vi "HGdynamicTest.vi"(0 "SceneObject in":refnum<vi>, 1 "data (can be any type)":string, 5 "Child 3":refnum<vi>, 7 "Angle Target":T1, 9 "Child 2":refnum<vi>, 11 "Child":refnum<vi>, 12 "Direction":enum16{"CW", "CCW"}(ring), 13 "Child 4":refnum<vi>) -> (2 "Angle":sgl, 3 "x*y":dbl, 4 "SceneNode out":refnum<vi>(3d-picture), 6 "number":dbl, 8 "number 2":dbl, 10 "number 3":dbl, 14 "number 5":dbl, 15 "number 4":dbl)   [LabVIEW 2020]
uses:
  Angle Target NEW type def.ctl
  <vilib>/picture/3D Picture Control/NI_3D Picture Control.lvlib
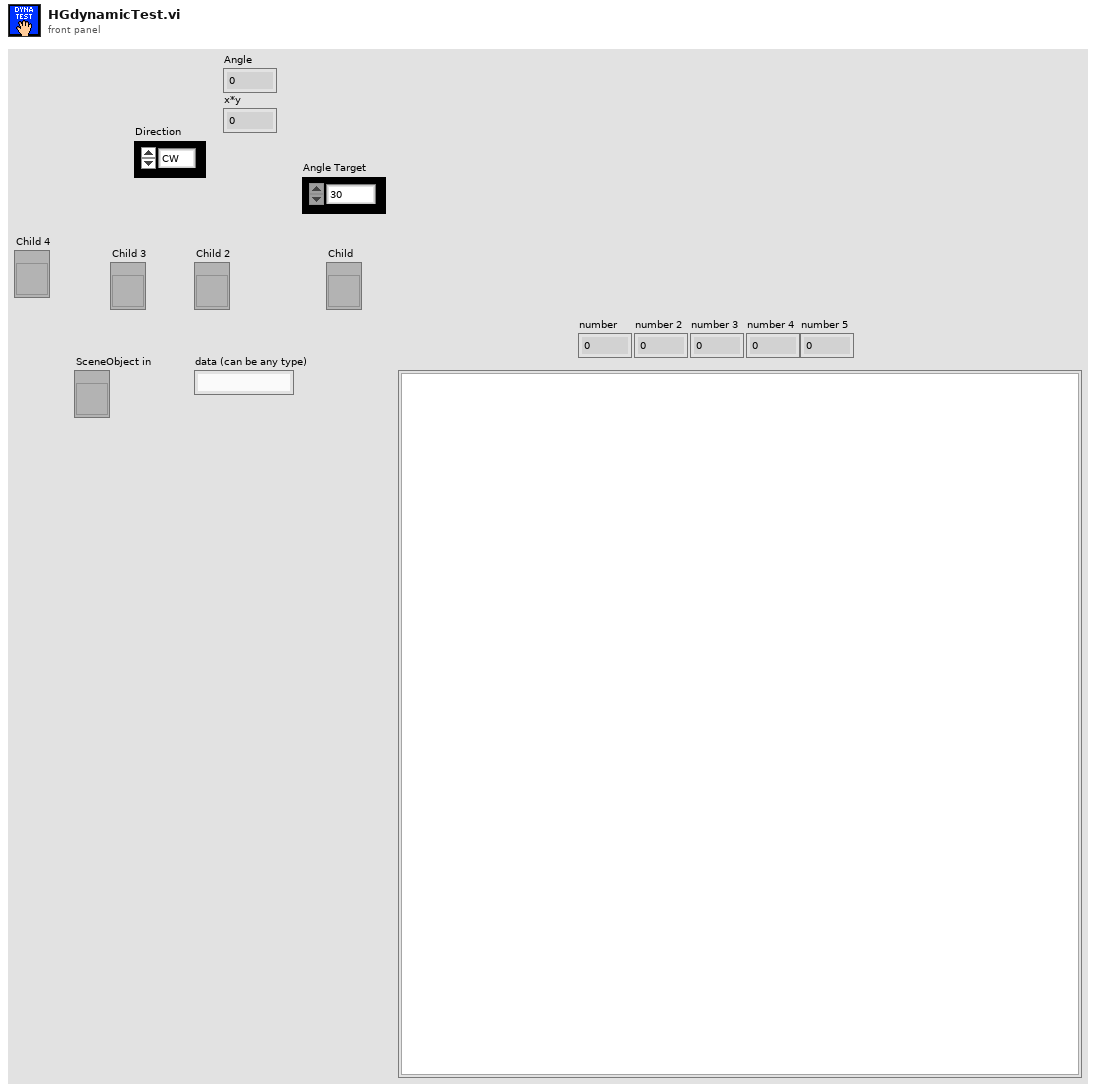
[diagram p1: front panel]
types:
  T1 = typedef "Angle Target NEW type def.ctl" = enum16{"30", "45", "60", "75", "90"}
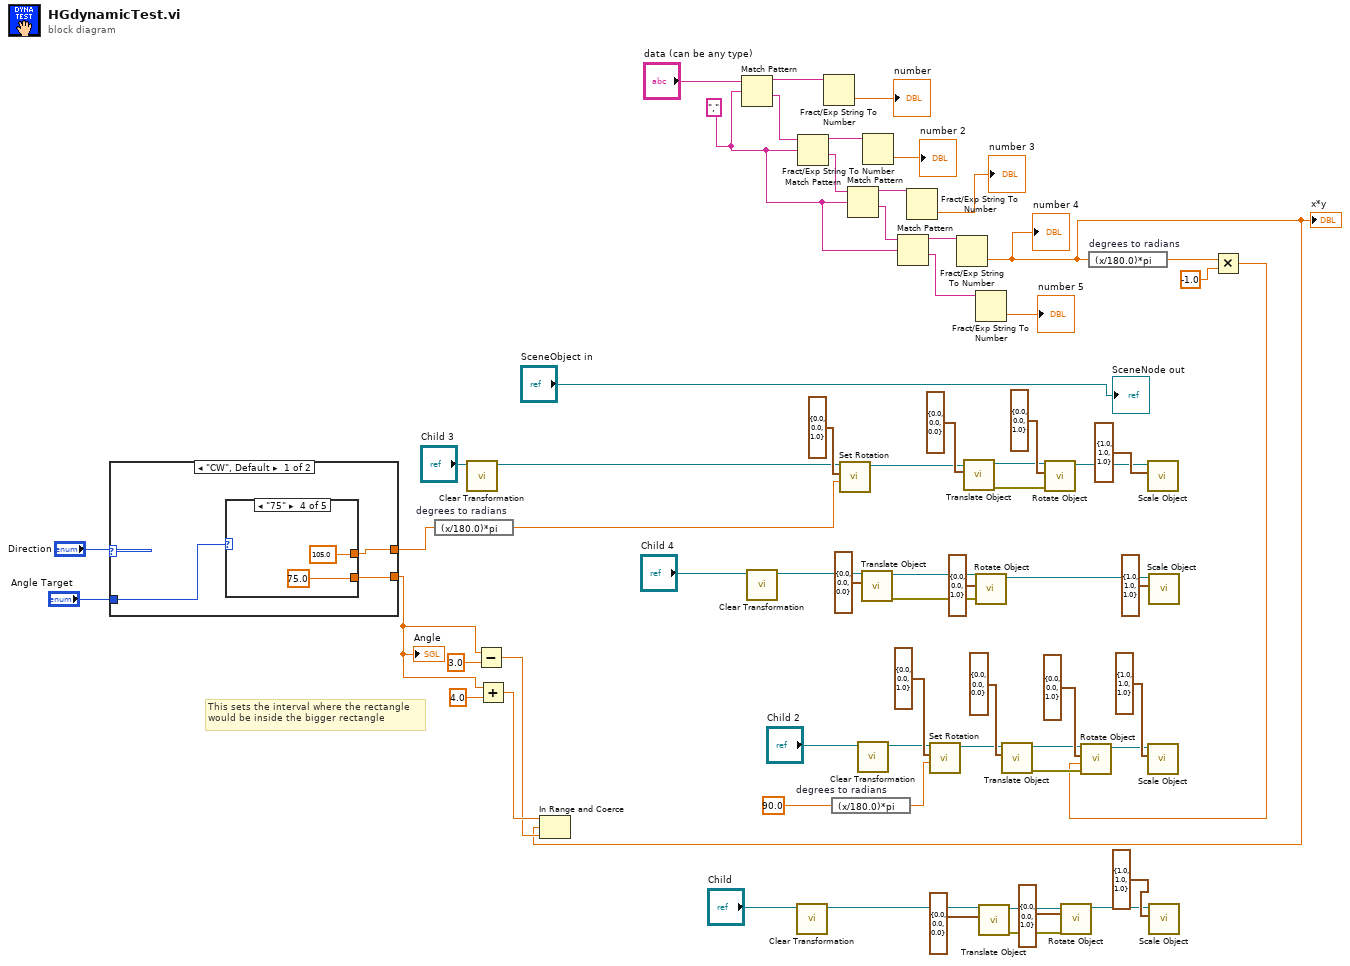
[diagram p0: block diagram]
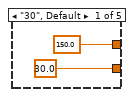
[diagram p2: hidden frame]
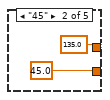
[diagram p3: hidden frame]
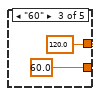
[diagram p4: hidden frame]
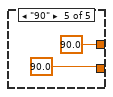
[diagram p5: hidden frame]
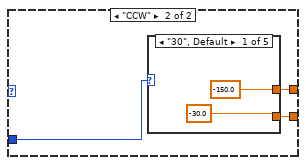
[diagram p6: hidden frame]
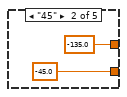
[diagram p7: hidden frame]
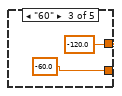
[diagram p8: hidden frame]
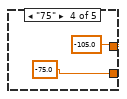
[diagram p9: hidden frame]
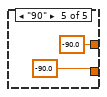
[diagram p10: hidden frame]
diagram:
  w5 = "," ("regular expression")
  # "This sets the interval where the rectangle \nwould be inside the bigger rectangle"
  n1 = case shown="\"CW\", Default" "Direction" {
    tunnel: [w69 w82] -> w14
    tunnel: [w68 w81] -> w8
    tunnel: "Angle Target" -> [w67 w80]
    frame "CW", Default {
      n2 = case shown="\"75\"" w67 {
        tunnel: [sgl 150.0 ("Angle") sgl 135.0 ("Angle") sgl 120.0 ("Angle") sgl 105.0 ("Angle") sgl 90.0 ("Angle")] -> w69
        tunnel: [30.0 45.0 60.0 75.0 90.0] -> w68
        frame "30", Default {
        }
        frame "45" {
        }
        frame "60" {
        }
        frame "75" {
        }
        frame "90" {
        }
      }
    }
    frame "CCW" {
      n3 = case shown="\"30\", Default" w80 {
        tunnel: [sgl -150.0 ("Angle") sgl -135.0 ("Angle") sgl -120.0 ("Angle") sgl -105.0 ("Angle") sgl -90.0 ("Angle")] -> w82
        tunnel: [-30.0 -45.0 -60.0 -75.0 -90.0] -> w81
        frame "30", Default {
        }
        frame "45" {
        }
        frame "60" {
        }
        frame "75" {
        }
        frame "90" {
        }
      }
    }
  }
  "Angle" <- w8
  n4 = expression code="(x/180.0)*pi" "degrees to radians"(w14) -> (w15:sgl)
  n5 = call <vilib>:"Clear Transformation.vi"("Object Refnum In"="Child 3") -> ("Object Refnum Out"=w13:refnum<vi>)  [unwired: 9 in, 1 out]
  n6 = Subtract(x=w8, y=sgl 3.0) -> (x-y=w11:dbl)
  n7 = Add(x=w8, y=sgl 4.0) -> (x+y=w12:dbl)
  n8 = Match Pattern(string="data (can be any type)", regular expression=w5) -> (before substring=w40:string, after substring=w39:string)  [unwired: 1 in, 2 out]
  n9 = call <vilib>:"Clear Transformation.vi"("Object Refnum In"="Child 4") -> ("Object Refnum Out"=w26:refnum<vi>)  [unwired: 9 in, 1 out]
  n10 = call <vilib>:"Clear Transformation.vi"("Object Refnum In"="Child") -> ("Object Refnum Out"=w44:refnum<vi>)  [unwired: 9 in, 1 out]
  n11 = Match Pattern(string=w39, regular expression=w5) -> (before substring=w41:string, after substring=w34:string)  [unwired: 1 in, 2 out]
  n12 = Fract/Exp String To Number(string=w40) -> (number=→"number":dbl)  [unwired: 3 in, 1 out]
  n13 = expression code="(x/180.0)*pi" "degrees to radians"(sgl 90.0 ("Angle")) -> (w19:sgl)
  n14 = call <vilib>:"Set Rotation.vi"("Angle"=w15, "Axis"=cluster{"X":sgl, "Y":sgl, "Z":sgl} {"X"=0.0, "Y"=0.0, "Z"=1.0}, "Scene Object"=w13) -> ("Rotated Scene Object"=w30:refnum<vi>)  [unwired: 7 in, 1 out]
  n15 = Match Pattern(string=w34, regular expression=w5) -> (before substring=w33:string, after substring=w6:string)  [unwired: 1 in, 2 out]
  n16 = call <vilib>:"Clear Transformation.vi"("Object Refnum In"="Child 2") -> ("Object Refnum Out"=w43:refnum<vi>)  [unwired: 9 in, 1 out]
  n17 = call <vilib>:"Translate Object.vi"("Translation"=cluster{"X":sgl, "Y":sgl, "Z":sgl} {"X"=0.0, "Y"=0.0, "Z"=0.0}, "Scene.Object In"=w26) -> ("error out"=w22:errorcluster, "Scene.Object Out"=w25:refnum<vi>)  [unwired: 8 in]
  n18 = Fract/Exp String To Number(string=w41) -> (number=→"number 2":dbl)  [unwired: 3 in, 1 out]
  n19 = Match Pattern(string=w6, regular expression=w5) -> (before substring=w4:string, after substring=w3:string)  [unwired: 1 in, 2 out]
  n20 = Fract/Exp String To Number(string=w33) -> (number=→"number 3":dbl)  [unwired: 3 in, 1 out]
  n21 = call <vilib>:"Set Rotation.vi"("Angle"=w19, "Axis"=cluster{"X":sgl, "Y":sgl, "Z":sgl} {"X"=0.0, "Y"=0.0, "Z"=1.0}, "Scene Object"=w43) -> ("Rotated Scene Object"=w42:refnum<vi>)  [unwired: 7 in, 1 out]
  n22 = Fract/Exp String To Number(string=w4) -> (number=w7:dbl)  [unwired: 3 in, 1 out]
  "number 4" <- w7
  "x*y" <- w7
  n23 = In Range and Coerce(upper limit=w12, x=w7, lower limit=w11) -> ()  [unwired: 2 out]
  n24 = call <vilib>:"Translate Object.vi"("Translation"=cluster{"X":sgl, "Y":sgl, "Z":sgl} {"X"=0.0, "Y"=0.0, "Z"=0.0}, "Scene.Object In"=w30) -> ("error out"=w53:errorcluster, "Scene.Object Out"=w52:refnum<vi>)  [unwired: 8 in]
  n25 = Fract/Exp String To Number(string=w3) -> (number=→"number 5":dbl)  [unwired: 3 in, 1 out]
  n26 = call <vilib>:"Rotate Object.vi"("error in (no error)"=w22, "Axis"=cluster{"X":sgl, "Y":sgl, "Z":sgl} {"X"=0.0, "Y"=0.0, "Z"=1.0}, "Scene.Object In"=w25) -> ("Scene.Object Out"=w24:refnum<vi>)  [unwired: 7 in, 1 out]
  n27 = call <vilib>:"Translate Object.vi"("Translation"=cluster{"X":sgl, "Y":sgl, "Z":sgl} {"X"=0.0, "Y"=0.0, "Z"=0.0}, "Scene.Object In"=w44) -> ("error out"=w47:errorcluster, "Scene.Object Out"=w46:refnum<vi>)  [unwired: 8 in]
  n28 = call <vilib>:"Translate Object.vi"("Translation"=cluster{"X":sgl, "Y":sgl, "Z":sgl} {"X"=0.0, "Y"=0.0, "Z"=0.0} ("Translation 2"), "Scene.Object In"=w42) -> ("error out"=w50:errorcluster, "Scene.Object Out"=w49:refnum<vi>)  [unwired: 8 in]
  n29 = call <vilib>:"Rotate Object.vi"("error in (no error)"=w53, "Axis"=cluster{"X":sgl, "Y":sgl, "Z":sgl} {"X"=0.0, "Y"=0.0, "Z"=1.0}, "Scene.Object In"=w52) -> ("Scene.Object Out"=w51:refnum<vi>)  [unwired: 7 in, 1 out]
  n30 = call <vilib>:"Rotate Object.vi"("error in (no error)"=w47, "Axis"=cluster{"X":sgl, "Y":sgl, "Z":sgl} {"X"=0.0, "Y"=0.0, "Z"=1.0}, "Scene.Object In"=w46) -> ("Scene.Object Out"=w45:refnum<vi>)  [unwired: 7 in, 1 out]
  n31 = expression code="(x/180.0)*pi" "degrees to radians"(w7) -> (w18:dbl)
  n32 = call <vilib>:"Scale Object.vi"("Scale"=cluster{"X":sgl, "Y":sgl, "Z":sgl} {"X"=1.0, "Y"=1.0, "Z"=1.0}, "Scene.Object In"=w51) -> ()  [unwired: 8 in, 2 out]
  n33 = call <vilib>:"Scale Object.vi"("Scale"=cluster{"X":sgl, "Y":sgl, "Z":sgl} {"X"=1.0, "Y"=1.0, "Z"=1.0}, "Scene.Object In"=w24) -> ()  [unwired: 8 in, 2 out]
  n34 = call <vilib>:"Scale Object.vi"("Scale"=cluster{"X":sgl, "Y":sgl, "Z":sgl} {"X"=1.0, "Y"=1.0, "Z"=1.0}, "Scene.Object In"=w45) -> ()  [unwired: 8 in, 2 out]
  n35 = Multiply(x=w18, y=sgl -1.0 ("Angle")) -> (x*y=w16:dbl)
  n36 = call <vilib>:"Rotate Object.vi"("error in (no error)"=w50, "Angle"=w16, "Axis"=cluster{"X":sgl, "Y":sgl, "Z":sgl} {"X"=0.0, "Y"=0.0, "Z"=1.0} ("Axis 2"), "Scene.Object In"=w49) -> ("Scene.Object Out"=w48:refnum<vi>)  [unwired: 6 in, 1 out]
  n37 = call <vilib>:"Scale Object.vi"("Scale"=cluster{"X":sgl, "Y":sgl, "Z":sgl} {"X"=1.0, "Y"=1.0, "Z"=1.0}, "Scene.Object In"=w48) -> ()  [unwired: 8 in, 2 out]
  "SceneNode out" <- "SceneObject in"
